vi "TCP Server Get Connections Info.vi"(8 "error in (no error)":errorcluster, 11 "TCP Server":refnum<class "JKI TCP Server.lvclass">) -> (0 "error out":errorcluster, 1 "Connections Info":T1[](array[typedef]), 2 "Number of Connections":u32, 3 "TCP Server out":refnum<class "JKI TCP Server.lvclass">, 5 "time running (s)":dbl)   [LabVIEW 2020, in "JKI TCP Server.lvclass"]
uses:
  JKI TCP Server.lvclass
  JKI TCP Server.lvclass/JKI TCP Server.ctl
  _Data Structures/TCP Server Public Connections Info Cluster.ctl
panel:
  # "Copyright © 2004-2008 JKI. All rights reserved.\n\nAuthor: Jim Kring [jim.kring@jameskring.com]\n\nThis library is provided \"AS IS\" ,WITHOUT WARRANTIES OR \nCONDITIONS OF ANY KIND, either express or implied.\n\nJames Kring, Inc. -- http://www.jameskring.com"
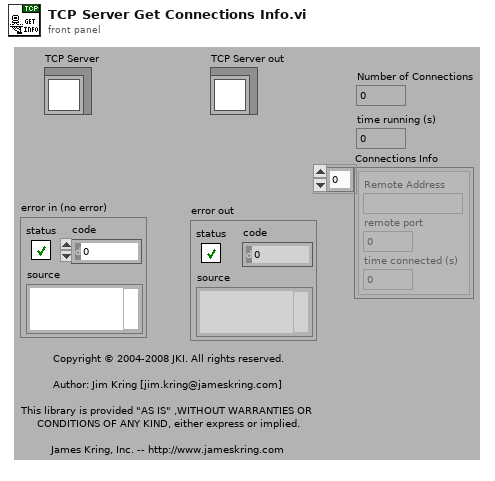
[diagram p1: front panel]
types:
  T1 = typedef "JKI TCP Server.lvclass/TCP Server Public Connections Info Cluster.ctl" = cluster{"Remote Address":string, "remote port":u16, "time connected (s)":dbl}
  T2 = typedef "JKI TCP Server.lvclass/TCP Server Data.ctl" = cluster{"Listener Info":T3, "Connection Process VI RefNums":refnum<vi>[], "dup connection IDs (for quick search)":refnum<k5>[], "Connections":T4[], "Connection Handler VI Path":path, "Handler Is Reentrant?":bool, "TCP Handler Instance RefNums":T5[], "TCP Handler VI RefNum":T5, "No. Connections":u32, "Max Connections":u32, "server start time":u32, "Additional Data":variant}
  T3 = typedef "JKI TCP Server.lvclass/TCP Server Listener Info Cluster.ctl" = cluster{"listener ID":refnum<k5>, "net address":u32, "port":u16, "Listener Process VI Refnum":refnum<vi>}
  T4 = typedef "JKI TCP Server.lvclass/TCP Server Connection Info Cluster.ctl" = cluster{"connection ID":refnum<k5>, "Remote Address":string, "remote port":u16, "connection start time":u32}
  T5 = typedef "JKI TCP Server.lvclass/TCP Server Handler RefNum.ctl" = refnum<vi>
  T6 = cluster{"Remote Address":string, "remote port":u16, dbl}
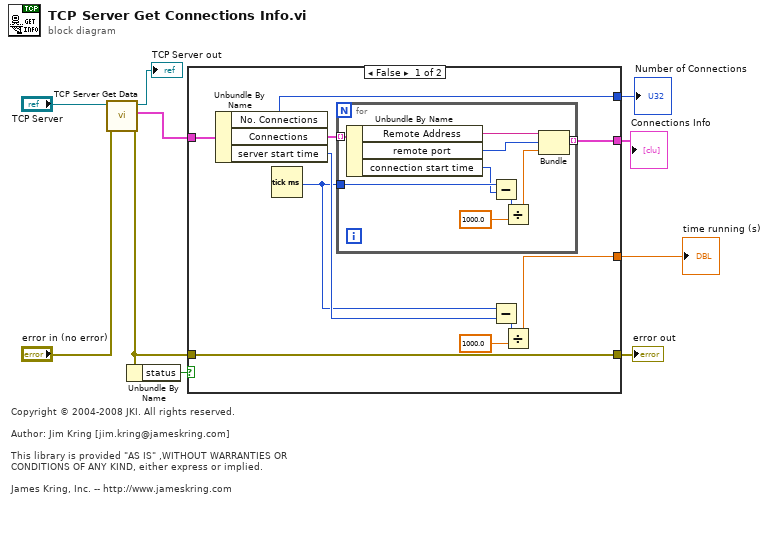
[diagram p0: block diagram]
diagram:
  # "Copyright © 2004-2008 JKI. All rights reserved.\n\nAuthor: Jim Kring [jim.kring@jameskring.com]\n\nThis library is provided \"AS IS\" ,WITHOUT WARRANTIES OR \nCONDITIONS OF ANY KIND, either express or implied.\n\nJames Kring, Inc. -- http://www.jameskring.com"
  n1 = call "TCP Server Get Data.vi"("error in (no error)"="error in (no error)", "RefNum"="TCP Server") -> ("error out"=w6:errorcluster, "Data out"=w8:T2, "dup RefNum"=→"TCP Server out":refnum<class "JKI TCP Server.lvclass">)  [unwired: 7 in]
  n2 = Unbundle By Name(w6) -> ("status"=w10:bool)
  n3 = case shown="False" w10 {
    tunnel: w6 -> [w19 w30]
    tunnel: [w19 w30] -> w9
    tunnel: w8 -> [w20 _]
    tunnel: [w16 _] -> w3
    tunnel: [w17 _] -> w2
    tunnel: [w11 _] -> w1
    frame False {
      n4 = Unbundle By Name(w20) -> ("No. Connections"=w16:u32, "Connections"=w18:T4[], "server start time"=w13:u32)
      n5 = Tick Count (ms)() -> (millisecond timer value=w12:u32)
      n6 = for {
        tunnel: w18 -> [w28] mode=indexing
        tunnel: [w29] -> w17 mode=indexing
        tunnel: w12 -> [w23]
        n7 = Unbundle By Name(w28) -> ("Remote Address"=w27:string, "remote port"=w26:u16, "connection start time"=w22:u32)
        n8 = Subtract(x=w23, y=w22) -> (x-y=w24:u32)
        n9 = Divide(x=w24, y=1000.0) -> (x/y=w21:dbl)
        n10 = Bundle("Remote Address"=w27, "remote port"=w26, w21) -> (w29:T6)  [unwired: 1 in]
      }
      n11 = Subtract(x=w12, y=w13) -> (x-y=w15:u32)
      n12 = Divide(x=w15, y=1000.0) -> (x/y=w11:dbl)
    }
    frame True {
      # "Error"
    }
  }
  "error out" <- w9
  "Number of Connections" <- w3
  "Connections Info" <- w2
  "time running (s)" <- w1
